vi "scope1.vi"(0 "instrument handle":refnum<k15>, 9 "TriggerMode":bool, 11 "error in":errorcluster) -> (6 "signal":T1(graph), 15 "error out":errorcluster)   [LabVIEW 2010]
doc: "Configures and acquires data from an NI-SCOPE high-speed digitizer.\n--------------------\n\nThis Express VI is configured as follows:\n\nDevice: ADC (PXI-5114)\nSample Rate (S/s): 10k\nRecord length: 2k\nAcquisition Mode: N Samples\nChannel 0\n - Range (V): 2\n - Offset (V): 0\n - Probe attenuation: 1\n - Coupling: \n - Input impedence: 1 \n - Bandwidth (Hz): 0\nChannel 1\n - Range (V): 2\n - Offset (V): 0\n - Probe attenuation: 1\n - Coupling: \n - Input impedence: 1 \n - Bandwidth (Hz): 0\nDigitalRTSI 4"
uses:
  <instrlib>/niScope/Controls/niScope timestamp type.ctl
  <instrlib>/niScope/Acquire/Fetch/niScope Multi Fetch Binary 8.vi
  glob1.vi
  <instrlib>/niScope/Configure/Trigger/niScope Configure Trigger Immediate.vi
  <instrlib>/niScope/Configure/Trigger/niScope Configure Trigger Digital.vi
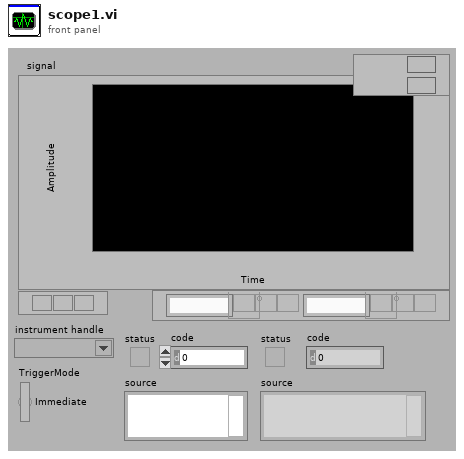
[diagram p1: front panel]
types:
  T1 = cluster{"relativeInitialX":dbl, "xIncrement":dbl, i16[][]}
  T2 = typedef "niScope timestamp type.ctl" = i32
  T3 = typedef "niScope vertical coupling.ctl" = i32
  T4 = cluster{"channel name":string, "input impedance":u32, "maximum input frequency":dbl, "vertical coupling":T3, "probe attenuation":dbl, "vertical range":dbl, "vertical offset":dbl, "channel enabled":bool}[]
  T5 = cluster{"enforce realtime":bool, "number of records":i32, "min sample rate":dbl, "reference position":dbl, "min record length":i32}
  T6 = typedef "niScope trigger slope.ctl" = i32
  T7 = typedef "niScope trigger source digital.ctl" = string
  T8 = cluster{"slope":T6, "source":T7, "holdoff":dbl, "delay":dbl}
  T9 = cluster{"channel name":bool, "input impedance":bool, "maximum input frequency":bool, "vertical coupling":bool, "probe attenuation":bool, "vertical range":bool, "vertical offset":bool, "channel enabled":bool}
  T10 = cluster{"enforce realtime":bool, "number of records":bool, "min sample rate":bool, "reference position":bool, "min record length":bool}
  T11 = cluster{"slope":bool, "source":bool, "holdoff":bool, "delay":bool}
  T12 = cluster{"actualSamples":i32, "absoluteInitialX":dbl, "relativeInitialX":dbl, "xIncrement":dbl, "offset":dbl, "gain":dbl, "reserved1":dbl, "reserved2":dbl}[]
  T13 = cluster{"actualSamples":i32, "absoluteInitialX":dbl, "relativeInitialX":dbl, "xIncrement":dbl, "offset":dbl, "gain":dbl, "reserved1":dbl, "reserved2":dbl}
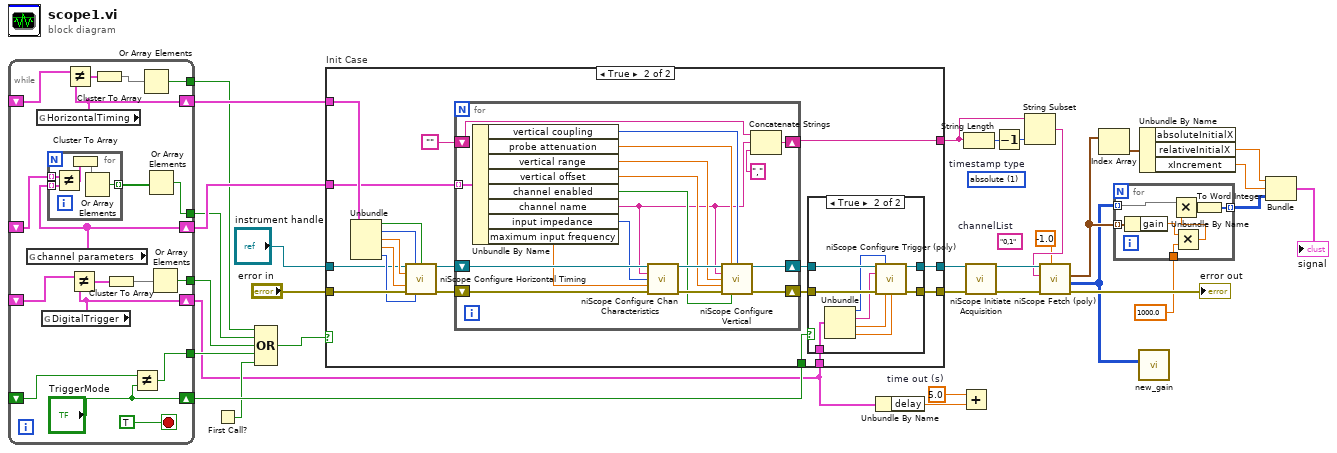
[diagram p0: block diagram]
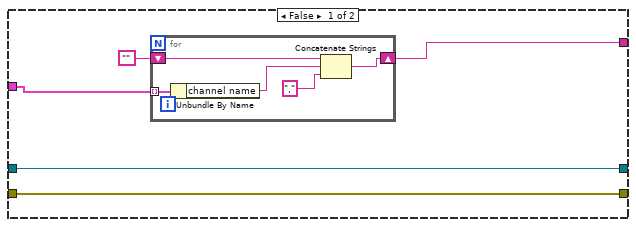
[diagram p2: hidden frame]
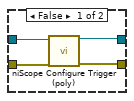
[diagram p3: hidden frame]
diagram:
  w3 = 5.0  # time out (s)
  (unwired) T2 1 items=["relative", "absolute"]  # timestamp type
  (unwired) "0,1"  # channelList
  n1 = while {
    shift-right: [w48] -> w21
    shift-left: _ -> [w49]
    shift-right: [w39] -> w20
    shift-left: _ -> [w40]
    shift-right: [w47] -> w4
    shift-left: _ -> [w46]
    tunnel: [w38] -> w18
    tunnel: [w37] -> w17
    tunnel: [w36] -> w16
    shift-right: ["TriggerMode"] -> w15
    shift-left: _ -> [w35]
    tunnel: [w33] -> w14
    stop <- TRUE stop-if-true
    n2 = global read "glob1.vi" "channel parameters"() -> (w39:T4)
    n3 = global read "glob1.vi" "HorizontalTiming"() -> (w48:T5)
    n4 = global read "glob1.vi" "DigitalTrigger"() -> (w47:T8)
    n5 = for {
      tunnel: [w54] -> w43 mode=indexing
      tunnel: w40 -> [w53] mode=indexing
      tunnel: w39 -> [w52] mode=indexing
      n6 = Not Equal?(x=w53, y=w52) -> (x != y?=w51:T9)
      n7 = Cluster To Array(cluster=w51) -> (array=w55:bool[])
      n8 = Or Array Elements(Boolean array=w55) -> (logical OR=w54:bool)
    }
    n9 = Not Equal?(x=w49, y=w48) -> (x != y?=w45:T10)
    n10 = Not Equal?(x=w46, y=w47) -> (x != y?=w44:T11)
    n11 = Cluster To Array(cluster=w45) -> (array=w42:bool[])
    n12 = Cluster To Array(cluster=w44) -> (array=w41:bool[])
    n13 = Not Equal?(x=w35, y="TriggerMode") -> (x != y?=w33:bool)
    n14 = Or Array Elements(Boolean array=w42) -> (logical OR=w38:bool)
    n15 = Or Array Elements(Boolean array=w43) -> (logical OR=w37:bool)
    n16 = Or Array Elements(Boolean array=w41) -> (logical OR=w36:bool)
  }
  n17 = First Call?() -> (First Call?: T/F=w13:bool)
  n18 = Compound Arithmetic op=OR(w18, w17, w16, w14, w13) -> (w19:bool)
  n19 = case "Init Case" shown="True" w19 {
    tunnel: "error in" -> [w60 w78]
    tunnel: [w60 w81] -> w32
    tunnel: [w59 w82] -> w29
    tunnel: w21 -> [_ w77]
    tunnel: w20 -> [w57 w68]
    tunnel: "instrument handle" -> [w59 w71]
    tunnel: w4 -> [_ w70]
    tunnel: w15 -> [_ w69]
    tunnel: [w56 w66] -> w10
    frame False {
      n20 = for {
        tunnel: w57 -> [w65] mode=indexing
        shift-right: [w63] -> w56
        shift-left: "" -> [w64]
        n21 = Unbundle By Name(w65) -> ("channel name"=w62:string)
        n22 = Concatenate Strings(w64, w62, ",") -> (w63:string)
      }
    }
    frame True {
      n23 = Unbundle(w77) -> ("enforce realtime"=w76:bool, "number of records"=w75:i32, "min sample rate"=w74:dbl, "reference position"=w73:dbl, "min record length"=w72:i32)
      n24 = call <instrlib>:"niScope Configure Horizontal Timing.vi"("instrument handle"=w71, "number of records"=w75, "enforce realtime"=w76, "min sample rate"=w74, "reference position"=w73, "error in"=w78, "min record length"=w72) -> ("instrument handle out"=w83:refnum<k15>, "error out"=w84:errorcluster)  [unwired: 7 in]
      n25 = for {
        shift-right: [w103] -> w79
        shift-left: w84 -> [w115]
        shift-right: [w102] -> w80
        shift-left: w83 -> [w114]
        tunnel: w68 -> [w111] mode=indexing
        shift-right: [w101] -> w66
        shift-left: "" -> [w100]
        n26 = Unbundle By Name(w111) -> ("vertical coupling"=w108:T3, "probe attenuation"=w107:dbl, "vertical range"=w106:dbl, "vertical offset"=w105:dbl, "channel enabled"=w104:bool, "channel name"=w99:string, "input impedance"=w109:u32, "maximum input frequency"=w110:dbl)
        n27 = call <instrlib>:"niScope Configure Chan Characteristics.vi"("instrument handle"=w114, "channels"=w99, "input impedance"=w109, "maximum input frequency"=w110, "error in"=w115) -> ("instrument handle out"=w113:refnum<k15>, "error out"=w112:errorcluster)  [unwired: 9 in]
        n28 = call <instrlib>:"niScope Configure Vertical.vi"("instrument handle"=w113, "probe attenuation"=w107, "vertical coupling"=w108, "channels"=w99, "vertical range"=w106, "vertical offset"=w105, "error in"=w112, "channel enabled"=w104) -> ("instrument handle out"=w102:refnum<k15>, "error out"=w103:errorcluster)  [unwired: 6 in]
        n29 = Concatenate Strings(w100, w99, ",") -> (w101:string)
      }
      n30 = case shown="True" w69 {
        tunnel: [w86 w97] -> w82
        tunnel: [w85 w96] -> w81
        tunnel: w80 -> [w88 w95]
        tunnel: w79 -> [w87 w94]
        tunnel: w70 -> [_ w89]
        frame False {
          n31 = call-poly <instrlib>:"niScope Configure Trigger (poly).vi"("instrument handle"=w88, "error in"=w87) -> ("instrument handle out"=w86:refnum<k15>, "error out"=w85:errorcluster)  [unwired: 12 in]
        }
        frame True {
          n32 = Unbundle(w89) -> ("slope"=w93:T6, "source"=w92:T7, "holdoff"=w91:dbl, "delay"=w90:dbl)
          n33 = call-poly <instrlib>:"niScope Configure Trigger (poly).vi"("instrument handle"=w95, "trigger slope"=w93, "trigger source"=w92, "error in"=w94, "trigger holdoff"=w91, "trigger delay"=w90) -> ("instrument handle out"=w97:refnum<k15>, "error out"=w96:errorcluster)  [unwired: 8 in]
        }
      }
    }
  }
  n34 = Unbundle By Name(w4) -> ("delay"=w2:dbl)
  n35 = Add(x=w3, y=w2) -> ()  [unwired: 1 out]
  n36 = String Length(string=w10) -> (length=w11:i32)
  n37 = call <instrlib>:"niScope Initiate Acquisition.vi"("instrument handle"=w29, "error in"=w32) -> ("instrument handle out"=w30:refnum<k15>, "error out"=w31:errorcluster)  [unwired: 12 in]
  n38 = Decrement(x=w11) -> (x-1=w12:i32)
  n39 = String Subset(string=w10, length (rest)=w12) -> (substring=w9:string)  [unwired: 1 in]
  n40 = call-poly <instrlib>:"niScope Fetch (poly).vi"("timeout"=-1.0, "error in"=w31, "channels"=w9, "instrument handle"=w30) -> ("error out"=→"error out":errorcluster, "wfm"=w5:i8[][], "wfm info"=w8:T12)  [unwired: 4 in, 1 out]
  n41 = Index Array(array=w8) -> (element=w28:T13)  [unwired: 1 in]
  n42 = for {
    tunnel: w5 -> [w121] mode=indexing
    tunnel: w8 -> [w122] mode=indexing
    tunnel: [w120] -> w7 mode=indexing
    tunnel: 1000.0 -> [w116]
    n43 = Unbundle By Name(w122) -> ("gain"=w118:dbl)
    n44 = Multiply(x=w118, y=w116) -> (x*y=w117:dbl)
    n45 = Multiply(x=w121, y=w117) -> (x*y=w119:dbl[])
    n46 = To Word Integer(number=w119) -> (16bit integer=w120:i16[])
  }
  n47 = call "new_gain.vi"("Array_in"=w5) -> ()  [unwired: 7 in]
  n48 = Unbundle By Name(w28) -> ("relativeInitialX"=w25:dbl, "xIncrement"=w27:dbl)  [unwired: 1 out]
  n49 = Bundle("relativeInitialX"=w25, "xIncrement"=w27, w7) -> (→"signal":T1)  [unwired: 1 in]
